vi "EditorPDF example.vi"() -> ()   [LabVIEW 2018]
uses:
  <vilib>/Simplicity AI/SAI_PDF_API/Classes/Context/Controls/SAI_PDF_Header-Footer (Simple).ctl
  <vilib>/Simplicity AI/SAI_PDF_API/Classes/Context/Controls/SAI_PDF_PDF Details.ctl
  <vilib>/Simplicity AI/SAI_PDF_API/Classes/Context/Controls/SAI_PDF_StdPageLayout.ctl
  <vilib>/Simplicity AI/SAI_PDF_API/Classes/Context/Controls/SAI_PDF_StdPageSize.ctl
  <vilib>/Simplicity AI/SAI_PDF_API/Classes/Context/Controls/SAI_PDF_Font.ctl
  <vilib>/Simplicity AI/SAI_PDF_API/Classes/Context/Controls/SAI_PDF_Font Encoding.ctl
  <vilib>/Simplicity AI/SAI_PDF_API/Classes/Context/Controls/SAI_PDF_Header-Footer Type.ctl
  <vilib>/Simplicity AI/SAI_PDF_API/Classes/Context/Controls/SAI_PDF_PDF Configuration.ctl
  <vilib>/Simplicity AI/SAI_PDF_API/Classes/Context/Controls/SAI_PDF_Type.ctl
  <vilib>/Simplicity AI/SAI_PDF_API/Classes/Context/Controls/SAI_PDF_Encryption Details.ctl
  <vilib>/Simplicity AI/SAI_PDF_API/Classes/Context/Controls/SAI_PDF_Encryption Strength.ctl
  <vilib>/Simplicity AI/SAI_PDF_API/Classes/Context/Controls/SAI_PDF_Encryption Permissions.ctl
  <vilib>/Simplicity AI/SAI_PDF_API/Classes/Context/Controls/SAI_PDF_Page Configuration.ctl
  <vilib>/Simplicity AI/SAI_PDF_API/Classes/Context/Controls/SAI_PDF_Page Layout Type.ctl
  <vilib>/Simplicity AI/SAI_PDF_API/Classes/Context/Controls/SAI_PDF_CustPageLayout.ctl
  <vilib>/Simplicity AI/SAI_PDF_API/Classes/Context/Controls/SAI_PDF_Margins.ctl
  <vilib>/Simplicity AI/SAI_PDF_API/Classes/Context/Methods/Public/Low Level/Add/SAI_PDF_Add Paragraph.vi
  <vilib>/Simplicity AI/SAI_PDF_API/Classes/Context/Context.lvclass
  <vilib>/Simplicity AI/SAI_PDF_API/SAI_PDF_Toolkit.lvlib
panel:
  in  "Font":T1={"Font"="Arial", "Size"=10, "Colour"=0, "Bold"=FALSE, "Italic"=FALSE, "Underline"=FALSE, "Strikethrough"=FALSE, "Font Encoding"=enum."Cp1252, WinANSI"}
  in  "error in (no error)":errorcluster
  in  "Standard Page":T3={"Page Size"=10, "Portrait (T:Yes)"=TRUE} {"Page Size" items=["LETTER", "NOTE", "LEGAL", "TABLOID", "EXECUTIVE", "POSTCARD", "A0", "A1", "A2", "A3", "A4", "A5", "A6", "A7", "A8", "A9", "A10", "B0", "B1", "B2", "B3", "B4", "B5", "B6", "B7", "B8", "B9", "B10", "ARCH_E", "ARCH_D", "ARCH_C", "ARCH_B", "ARCH_A", "FLSA", "FLSE", "HALFLETTER", "_11X17", "ID_1", "ID_2", "ID_3", "LEDGER", "CROWN_QUARTO", "LARGE_CROWN_QUARTO", "DEMY_QUARTO", "ROYAL_QUARTO", "CROWN_OCTAVO", "LARGE_CROWN_OCTAVO", "DEMY_OCTAVO", "ROYAL_OCTAVO", "SMALL_PAPERBACK", "PENGUIN_SMALL_PAPERBACK", "PENGUIN_LARGE_PAPERBACK"]}
  in  "PDF Details":T5={"Title"="UserCustom1", "Subject"="", "Keywords"="", "Author"="UserName", "Creator"="Acromass Editor"}
  in  "Header/Footer":T6={"Header Title"="UserCustom2", "Header Left"="", "Header Right"="Acromass", "Footer Title"="DataSource"}
  # "(Cp1252)"
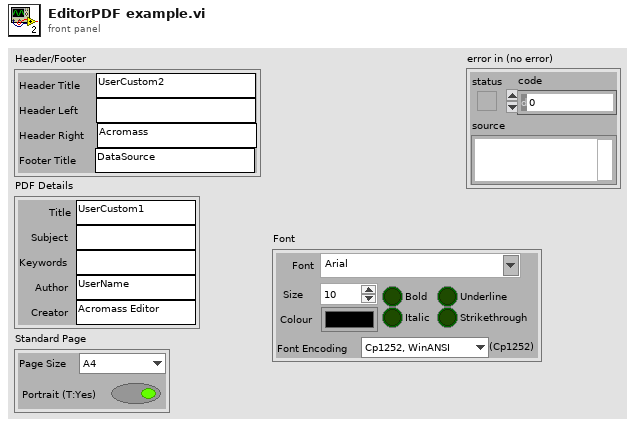
[diagram p1: front panel]
types:
  T1 = typedef "SAI_PDF_Toolkit.lvlib/Context.lvclass/SAI_PDF_Font.ctl" = cluster{"Font":string, "Size":i32, "Colour":u32, "Bold":bool, "Italic":bool, "Underline":bool, "Strikethrough":bool, "Font Encoding":T2}
  T2 = typedef "SAI_PDF_Toolkit.lvlib/Context.lvclass/SAI_PDF_Font Encoding.ctl" = enum16{"Cp1252, WinANSI", "IdentityH", "IdentityV", "Cp1250", "Cp1257", "MacRoman"}
  T3 = typedef "SAI_PDF_Toolkit.lvlib/Context.lvclass/SAI_PDF_StdPageLayout.ctl" = cluster{"Page Size":T4, "Portrait (T:Yes)":bool}
  T4 = typedef "SAI_PDF_Toolkit.lvlib/Context.lvclass/SAI_PDF_StdPageSize.ctl" = i32
  T5 = typedef "SAI_PDF_Toolkit.lvlib/Context.lvclass/SAI_PDF_PDF Details.ctl" = cluster{"Title":string, "Subject":string, "Keywords":string, "Author":string, "Creator":string}
  T6 = typedef "SAI_PDF_Toolkit.lvlib/Context.lvclass/SAI_PDF_Header-Footer (Simple).ctl" = cluster{"Header Title":string, "Header Left":string, "Header Right":string, "Footer Title":string}
  T7 = typedef "SAI_PDF_Toolkit.lvlib/Context.lvclass/SAI_PDF_Page Configuration.ctl" = cluster{"Page Layout Type":T8, "Standard Page Layout":T3, "Custom Page Layout":T9, "Margin":T10}
  T8 = typedef "SAI_PDF_Toolkit.lvlib/Context.lvclass/SAI_PDF_Page Layout Type.ctl" = enum16{"Standard", "Custom"}
  T9 = typedef "SAI_PDF_Toolkit.lvlib/Context.lvclass/SAI_PDF_CustPageLayout.ctl" = cluster{"X (mm)":sgl, "y (mm)":sgl}
  T10 = typedef "SAI_PDF_Toolkit.lvlib/Context.lvclass/SAI_PDF_Margins.ctl" = cluster{"Left":sgl, "Right":sgl, "Top":sgl, "Bottom":sgl}
  T11 = typedef "SAI_PDF_Toolkit.lvlib/Context.lvclass/SAI_PDF_Type.ctl" = i32
  T12 = typedef "SAI_PDF_Toolkit.lvlib/Context.lvclass/SAI_PDF_PDF Configuration.ctl" = cluster{"PDF Type":T11, "PDF Details":T5, "Encrypt? (F:No)":bool, "Encryption Details":T13}
  T13 = typedef "SAI_PDF_Toolkit.lvlib/Context.lvclass/SAI_PDF_Encryption Details.ctl" = cluster{"Strength":T14, "User Password":string, "Owner Password":string, "Permissions":T15[]}
  T14 = typedef "SAI_PDF_Toolkit.lvlib/Context.lvclass/SAI_PDF_Encryption Strength.ctl" = enum32{"Standard 40 bit", "Standard 128 bit", "AES 128 bit"}
  T15 = typedef "SAI_PDF_Toolkit.lvlib/Context.lvclass/SAI_PDF_Encryption Permissions.ctl" = i32
  T16 = typedef "SAI_PDF_Toolkit.lvlib/Context.lvclass/SAI_PDF_Header-Footer Type.ctl" = enum16{"None", "Simple", "Custom"}
  T17 = cluster{"Header/Footer Type":T16, "Header/Footer":T6}
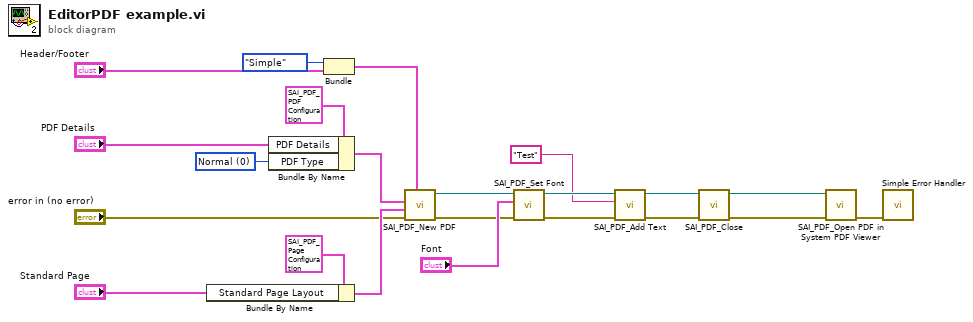
[diagram p0: block diagram]
diagram:
  w17 = T11 0 items=["Normal", "PDF_A_1b"] ("PDF Type")
  n1 = Bundle By Name(cluster=T7 {"Page Layout Type"=enum."Standard", "Standard Page Layout"={"Page Size"=10, "Portrait (T:Yes)"=TRUE}, "Custom Page Layout"={"X (mm)"=0.0, "y (mm)"=0.0}, "Margin"={"Left"=40.0, "Right"=40.0, "Top"=65.0, "Bottom"=55.0}} ("Page Configuration"), "Standard Page Layout"="Standard Page") -> (w13:T7)
  n2 = Bundle By Name(cluster=T12 {"PDF Type"=0, "PDF Details"={"Title"="", "Subject"="", "Keywords"="", "Author"="Simplicity AI", "Creator"="Simplicity AI PDF API"}, "Encrypt? (F:No)"=FALSE, "Encryption Details"={"Strength"=enum."Standard 128 bit", "User Password"="", "Owner Password"="", "Permissions"=[]}} ("PDF Configuration"), "PDF Details"="PDF Details", "PDF Type"=w17) -> (w16:T12)
  n3 = Bundle("Header/Footer Type"=SAI_PDF_Header-Footer_Type."Simple", "Header/Footer"="Header/Footer") -> (w20:T17)  [unwired: 1 out]
  n4 = call <vilib>:"SAI_PDF_New PDF.vi"("Header/Footer Configuration"=w20, "error in (no error)"="error in (no error)", "Page Configuration"=w13, "PDF Configuration"=w16) -> ("error out"=w9:errorcluster, "Context Out"=w10:refnum<class "Context.lvclass">)  [unwired: 5 in, 1 out]
  n5 = call <vilib>:"SAI_PDF_Set Font.vi"("error in"=w9, "Font"="Font", "Context In"=w10) -> ("error out"=w7:errorcluster, "Context Out"=w8:refnum<class "Context.lvclass">)  [unwired: 7 out]
  n6 = call-poly <vilib>:"SAI_PDF_Add Text.vi"("error in"=w7, "Text"="Test", "Context In"=w8) -> ("error out"=w6:errorcluster, "Context Out"=w5:refnum<class "Context.lvclass">)  [unwired: 1 in, 6 out]
  n7 = call <vilib>:"SAI_PDF_Close.vi"("error in"=w6, "Context In"=w5) -> ("error out"=w1:errorcluster, "Path"=w2:path)  [unwired: 8 in]
  n8 = call <vilib>:"SAI_PDF_Open PDF in System PDF Viewer.vi"("error in"=w1, "Path"=w2) -> ("error out"=w3:errorcluster)  [unwired: 9 out]
  n9 = call <vilib>:"Simple Error Handler.vi"("error in (no error)"=w3) -> ()  [unwired: 1 in, 8 out]
